vi "Group Check - CSM.vi"(8 "Matched Previous?":bool, 10 "Cross CSM Data (In)":T1={"Name (\"\" to Use UUID)"="", "Current State"="", "Arguments"="", "Source Message"={"‘State"="", "’Arguments"="", "’Error"={"status"=FALSE, "code"=0, "source"=""}}, "Source Module"="", "Complete(T)/Start(F)"=FALSE, "LogType"=enum."State Change", "Time Stamp"=timestamp(0 s since 1904-01-01)}, 11 "GlobalLogFilter.lvclass":refnum<class "LogFilter.lvclass">) -> (0 "Matched? (Dup)":bool, 2 "Cross CSM Data":T1={"Name (\"\" to Use UUID)"="", "Current State"="", "Arguments"="", "Source Message"={"‘State"="", "’Arguments"="", "’Error"={"status"=FALSE, "code"=0, "source"=""}}, "Source Module"="", "Complete(T)/Start(F)"=FALSE, "LogType"=enum."State Change", "Time Stamp"=timestamp(0 s since 1904-01-01)}, 3 "GlobalLogFilter.lvclass (Dup)":refnum<class "LogFilter.lvclass">)   [LabVIEW 2017, in "Communicable State Machine.lvlib" / "LogFilter.lvclass"]
doc: "### Group Check - CSM.vi\n\n-- <b>Controls</b> --\n- <b>Matched Previous?</b>:\n- <b>Cross CSM Data (in)</b>:\n- <b>GlobalLogFilter.lvclass</b>:\n\n-- <b>Indicators</b> --\n- <b>Matched? (dup)</b>:\n- <b>Cross CSM Data</b>:\n- <b>GlobalLogFilter.lvclass (dup)</b>:"
uses:
  LogFilter.lvclass
  Typedef/_CSM_GlobalLog_MSG.ctl
  Typedef/_CSM_Response Source Message.ctl
  Typedef/_CSM_GlobalLog_MSG_TYPE.ctl
  LogFilter.lvclass/LogFilter.ctl
  Communicable State Machine.lvlib
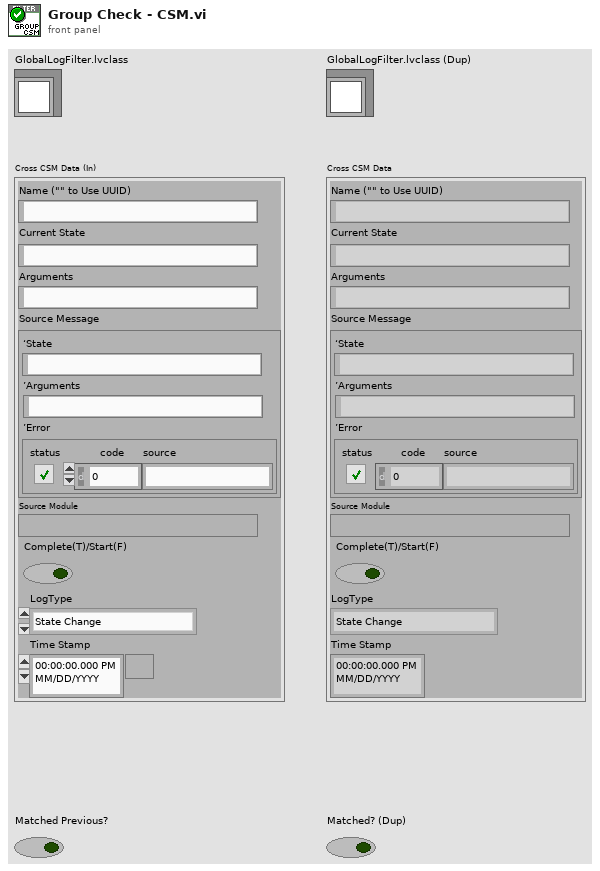
[diagram p1: front panel]
types:
  T1 = typedef "Communicable State Machine.lvlib/_CSM_GlobalLog_MSG.ctl" = cluster{"Name (\"\" to Use UUID)":string, "Current State":string, "Arguments":string, "Source Message":T2, "Source Module":string, "Complete(T)/Start(F)":bool, "LogType":T3, "Time Stamp":timestamp}
  T2 = typedef "Communicable State Machine.lvlib/_CSM_Response Source Message.ctl" = cluster{"‘State":string, "’Arguments":string, "’Error":errorcluster}
  T3 = typedef "Communicable State Machine.lvlib/_CSM_GlobalLog_MSG_TYPE.ctl" = enum16{"User Log", "State Change", "Status", "Interrupt", "Register", "Unregister", "Error Log", "Module Created", "Module Destroyed", "Async Message", "No-Rep Async Message", "Sync Message", "AsyncMsg Complete", "SyncMsg Complete"}
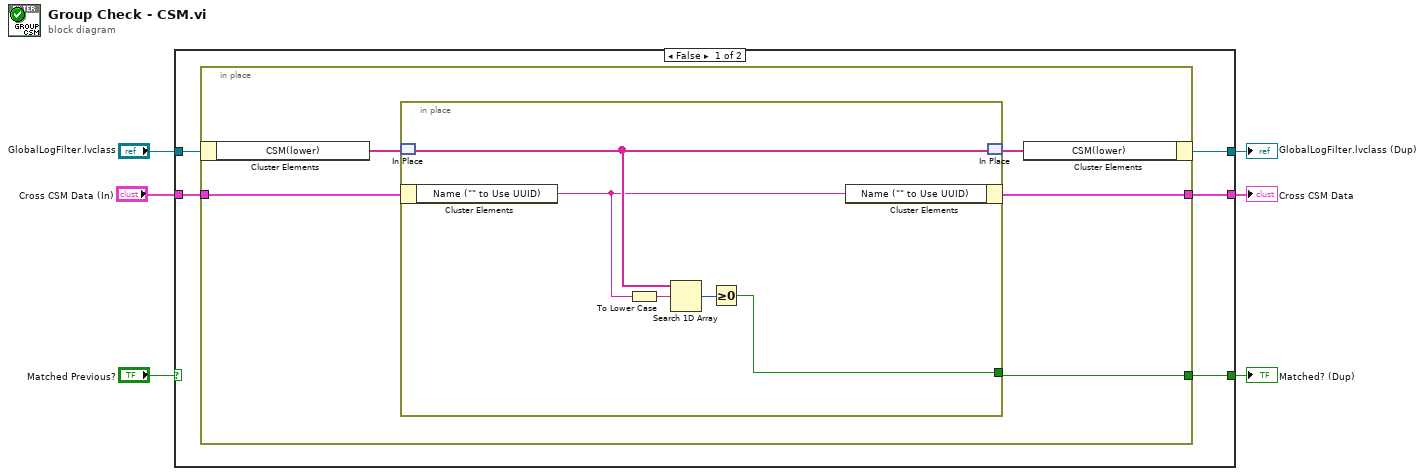
[diagram p0: block diagram]
diagram:
  n1 = case shown="False" "Matched Previous?" {
    selector: "Matched Previous?" -> [_ w23]
    tunnel: [w10 w24] -> w5
    tunnel: "Cross CSM Data (In)" -> [w11 w24]
    tunnel: [w9 w23] -> w3
    tunnel: [w7 w22] -> w2
    tunnel: "GlobalLogFilter.lvclass" -> [w8 w22]
    frame False {
      n2 = in-place {
        in-place-border: w11 -> [w16]
        in-place-border: [w15] -> w10
        in-place-border: [w14] -> w9
        n3 = in-place-cluster #1(w8) -> ("CSM(lower)"=w13:string[])
        n4 = in-place {
          in-place-border: [w20] -> w14
          n5 = in-place-match #2(w13) -> (w19:string[])
          n6 = in-place-cluster #3(w16) -> ("Name (\"\" to Use UUID)"=w18:string)
          n7 = To Lower Case(string=w18) -> (all lower case string=w17:string)
          n8 = Search 1D Array(1D array=w19, element=w17) -> (index of element=w21:i32)  [unwired: 1 in]
          n9 = Greater Or Equal To 0?(x=w21) -> (x >= 0?=w20:bool)
          n10 = in-place-cluster #3("Name (\"\" to Use UUID)"=w18) -> (w15:T1)
          n11 = in-place-match #2(w19) -> (w12:string[])
        }
        n12 = in-place-cluster #1("CSM(lower)"=w12) -> (w7:refnum<class "LogFilter.lvclass">)
      }
    }
    frame True {
    }
  }
  "Cross CSM Data" <- w5
  "Matched? (Dup)" <- w3
  "GlobalLogFilter.lvclass (Dup)" <- w2
